vi "HEWH Purge Time Adjustment.vi"(11 "Purge Time (Seconds) in":T1 format="%.2f") -> (3 "Purge Time (Seconds) out":T1 format="%.2f")   [LabVIEW 2016]
uses:
  Utility/Custom Pallet Controls/Custom Pallet DBL.ctl
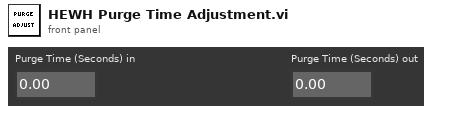
[diagram p1: front panel]
types:
  T1 = typedef "Custom Pallet DBL.ctl" = dbl
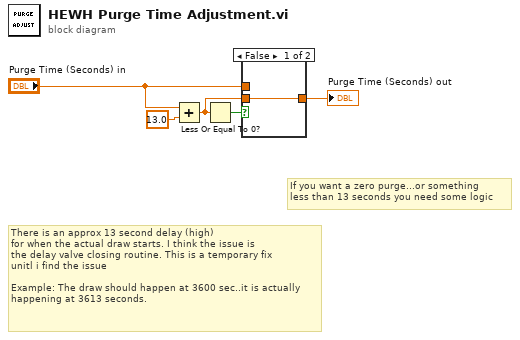
[diagram p0: block diagram]
diagram:
  # "If you want a zero purge...or something \nless than 13 seconds you need some logic"
  # "There is an approx 13 second delay (high) \nfor when the actual draw starts. I think the issue is \nthe delay valve closing routine. This is a temporary fix\nunitl i find the issue\n\nExample: The draw should happen at 3600 sec..it is actually\nhappening at 3613 seconds."
  n1 = Add(x="Purge Time (Seconds) in", y=T1 13.0) -> (x+y=w1:T1)
  n2 = Less Or Equal To 0?(x=w1) -> (x <= 0?=w4:bool)
  n3 = case shown="False" w4 {
    tunnel: [w6 w7] -> w3
    tunnel: w1 -> [w6 _]
    tunnel: "Purge Time (Seconds) in" -> [_ w7]
    frame False {
    }
    frame True {
    }
  }
  "Purge Time (Seconds) out" <- w3
